vi "Write Host IP Address.vi"(8 "error in (no error)":errorcluster, 10 "Host IP Address":string, 11 "PF_API in":refnum<class "PF_API.lvclass">) -> (0 "error out":errorcluster, 3 "PF_API out":refnum<class "PF_API.lvclass">)   [LabVIEW 2019, in "PF_API.lvclass"]
uses:
  PF_API.lvclass
  PF_API.lvclass/PF_API.ctl
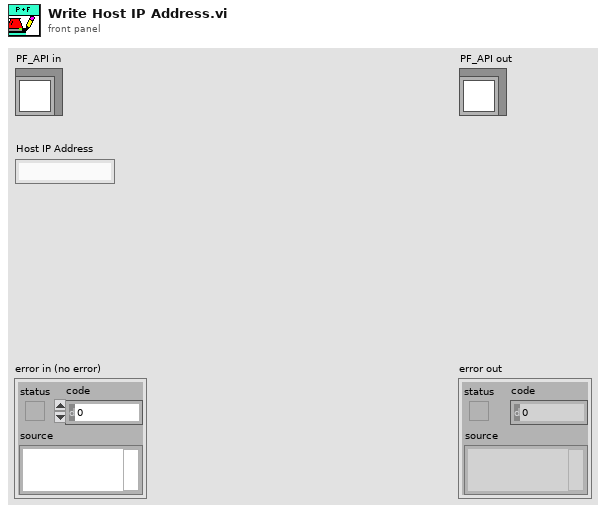
[diagram p1: front panel]
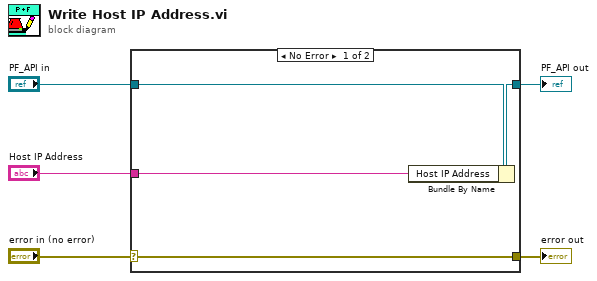
[diagram p0: block diagram]
diagram:
  n1 = case shown="No Error" "error in (no error)" {
    selector: "error in (no error)" -> [w9 w10]
    tunnel: [w9 w10] -> w4
    tunnel: [w7 w11] -> w2
    tunnel: "PF_API in" -> [w8 w11]
    tunnel: "Host IP Address" -> [w6 _]
    frame No Error {
      n2 = Bundle By Name(cluster=w8, "Host IP Address"=w6) -> (w7:refnum<class "PF_API.lvclass">)
    }
    frame Error {
    }
  }
  "error out" <- w4
  "PF_API out" <- w2
